vi "Read Task Hierarchy.vi"(8 "error in (no error)":errorcluster, 11 "Composite Map Task in":refnum<class "Composite Map Task.lvclass">) -> (0 "error out":errorcluster, 2 "Task Hierarchy":i64=-1, 3 "Composite Map Task out":refnum<class "Composite Map Task.lvclass">)   [LabVIEW 2022 SP3, in "Composite Map Task.lvclass"]
uses:
  Composite Map Task.lvclass
  Composite Map Task.lvclass/Composite Map Task.ctl
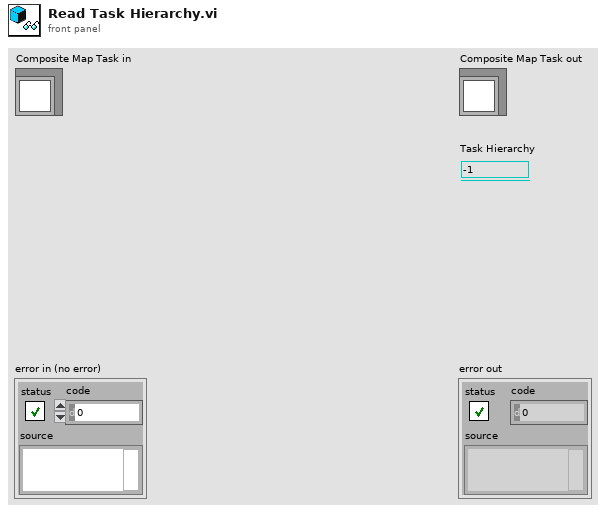
[diagram p1: front panel]
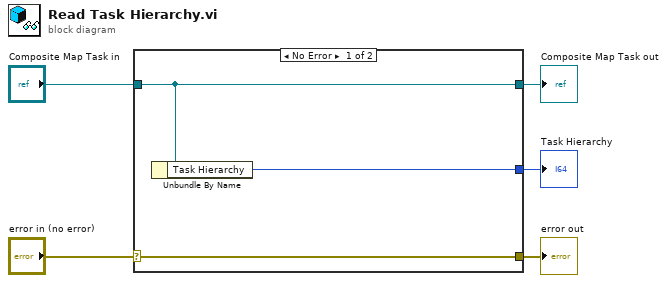
[diagram p0: block diagram]
diagram:
  n1 = case shown="No Error" "error in (no error)" {
    selector: "error in (no error)" -> [w8 w9]
    tunnel: [w8 w9] -> w4
    tunnel: [w7 w10] -> w2
    tunnel: "Composite Map Task in" -> [w7 w10]
    tunnel: [w6 _] -> w1
    frame No Error {
      n2 = Unbundle By Name(w7) -> ("Task Hierarchy"=w6:i64)
    }
    frame Error {
    }
  }
  "error out" <- w4
  "Composite Map Task out" <- w2
  "Task Hierarchy" <- w1
